vi "Replase ALR_RESETs.vi"(8 "error in (no error)":errorcluster, 9 "Reset":bool, 10 "Index":i32[](array[numeric]), 11 "ALR_ON_OFF":refnum<data-value>) -> (0 "error out":errorcluster, 3 "ALR_ON_OFF out":refnum<data-value>)   [LabVIEW 2019, in "Alarms.lvlib"]
uses:
  Alarms.lvlib
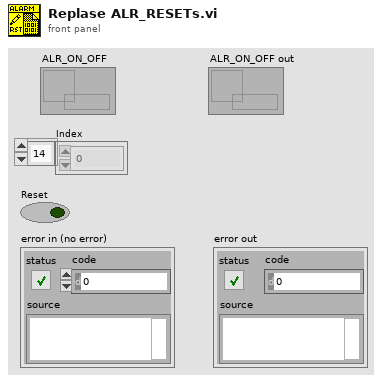
[diagram p1: front panel]
types:
  T1 = cluster{"ALR_ON":bool[], "ALR_OFF":bool[], "ALR_reset":bool[], "ALR_check":bool[], "ALR_block":bool[], "ALR_Ack":bool[]}
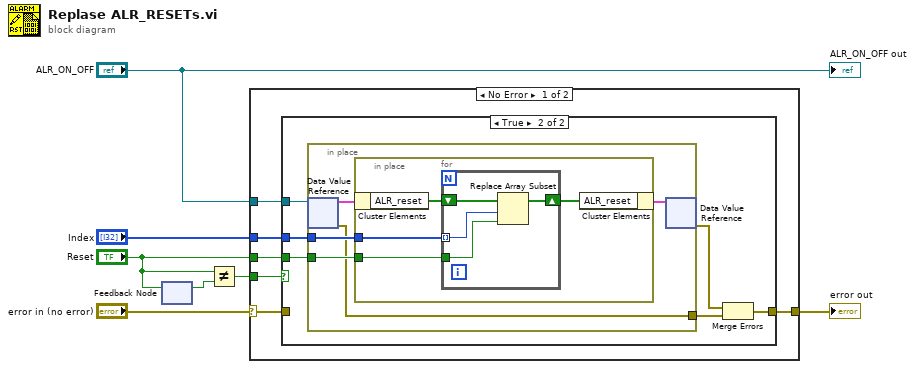
[diagram p0: block diagram]
diagram:
  n1 = feedback #1() -> (w4:bool)  [unwired: 1 in]
  n2 = feedback-in #1("Reset") -> ()
  n3 = Not Equal?(x="Reset", y=w4) -> (x != y?=w2:bool)
  n4 = case shown="No Error" "error in (no error)" {
    selector: "error in (no error)" -> [w9 w34]
    tunnel: "Index" -> [w13 _]
    tunnel: [w10 w34] -> w6
    tunnel: "ALR_ON_OFF" -> [w12 _]
    tunnel: "Reset" -> [w11 _]
    tunnel: w2 -> [w8 _]
    frame No Error {
      n5 = case shown="True" w8 {
        tunnel: w13 -> [_ w20]
        tunnel: w12 -> [_ w19]
        tunnel: w11 -> [_ w18]
        tunnel: [w14 w15] -> w10
        tunnel: w9 -> [w14 _]
        frame False {
        }
        frame True {
          n6 = in-place {
            in-place-border: w20 -> [w24]
            in-place-border: w18 -> [w23]
            in-place-border: [w21] -> w16
            n7 = in-place-dvr #2(w19) -> (w25:T1, w21:errorcluster)
            n8 = in-place {
              in-place-border: w24 -> [w28]
              in-place-border: w23 -> [w27]
              n9 = in-place-cluster #3(w25) -> ("ALR_reset"=w29:bool[])
              n10 = for {
                tunnel: w28 -> [w32] mode=indexing
                tunnel: w27 -> [w31]
                shift-right: [w30] -> w26
                shift-left: w29 -> [w33]
                n11 = Replace Array Subset(array=w33, new element=w31, index=w32) -> (w30:bool[])
              }
              n12 = in-place-cluster #3("ALR_reset"=w26) -> (w22:T1)
            }
            n13 = in-place-dvr #2(w22) -> (w17:errorcluster)  [unwired: 1 out]
          }
          n14 = Merge Errors(w17, w16) -> (w15:errorcluster)
        }
      }
    }
    frame Error {
    }
  }
  "error out" <- w6
  "ALR_ON_OFF out" <- "ALR_ON_OFF"
